vi "FGV_Dictionnaire.vi"(6 "FichierDictionnaire":path, 7 "Command":T3, 8 "error in (no error)":errorcluster, 9 "Dictionnaire In":T1, 10 "Chaîne":string, 11 "Clé":string) -> (0 "error out":errorcluster, 1 "Dictionnaire Out":T1, 3 "Traduction":string)   [LabVIEW 2011]
uses:
  EnumCommandDictionnaire.ctl
  Dictionnaire.ctl
  CleValeur.ctl
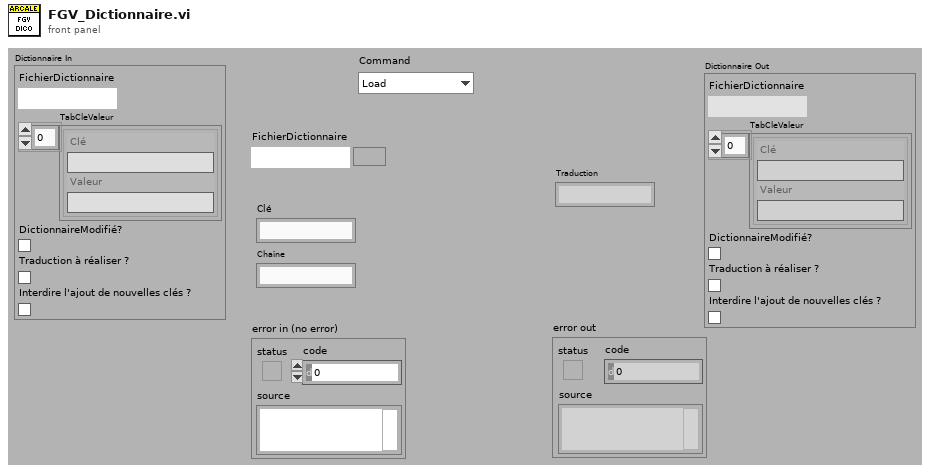
[diagram p1: front panel]
types:
  T1 = typedef "Dictionnaire.ctl" = cluster{"FichierDictionnaire":path, "TabCleValeur":T2[], "DictionnaireModifié?":bool, "Traduction à réaliser ?":bool, "Interdire l'ajout de nouvelles clés ?":bool}
  T2 = typedef "CleValeur.ctl" = cluster{"Clé":string, "Valeur":string}
  T3 = typedef "EnumCommandDictionnaire.ctl" = enum16{"Load", "Translate", "Save", "GetDico", "Set : A traduire = Vrai", "Set : A Traduire = Faux", "SetDico"}
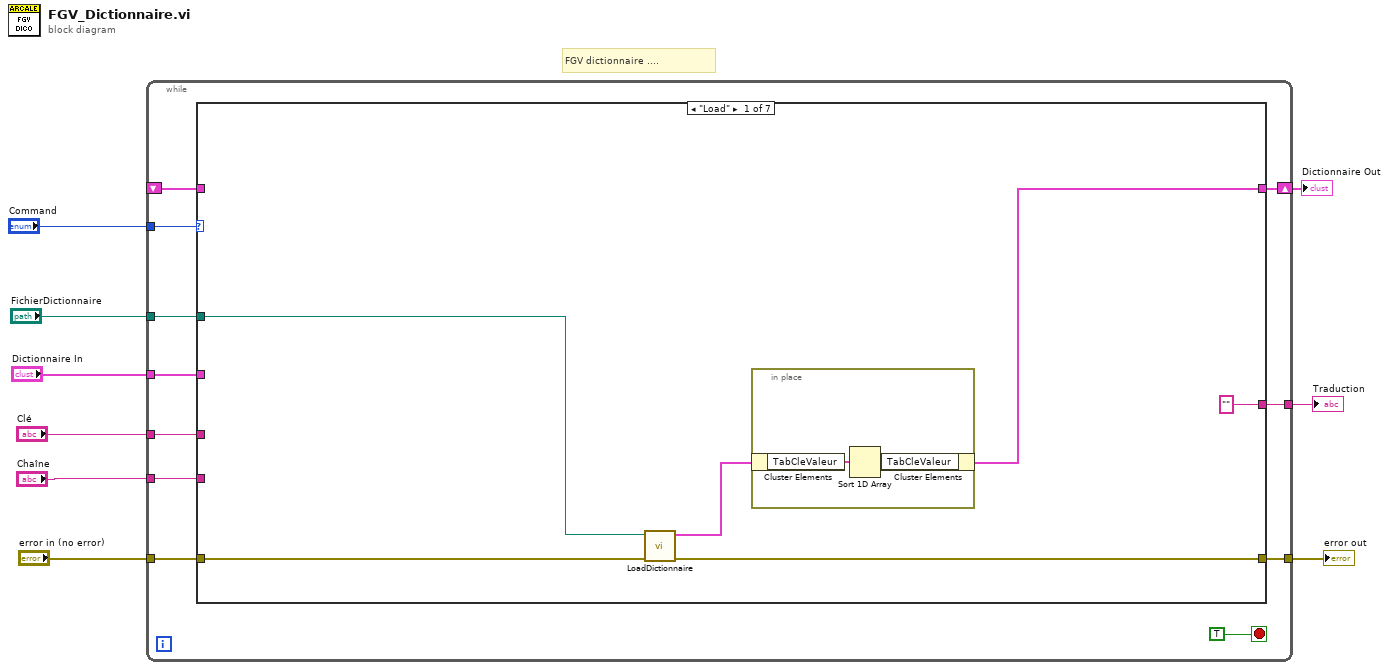
[diagram p0: block diagram]
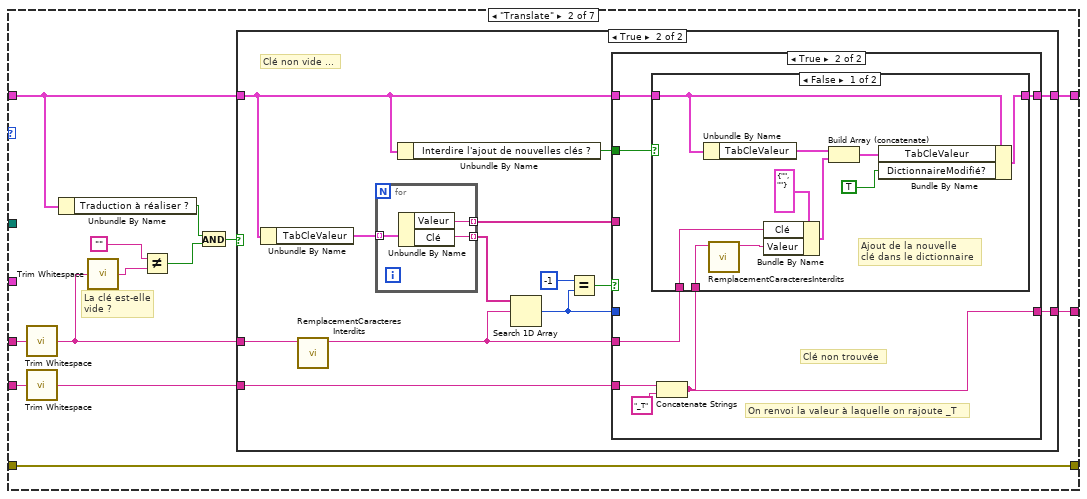
[diagram p2: hidden frame]
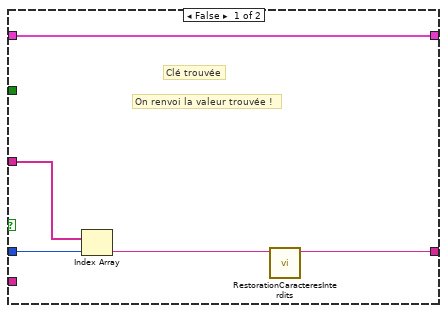
[diagram p4: hidden frame]
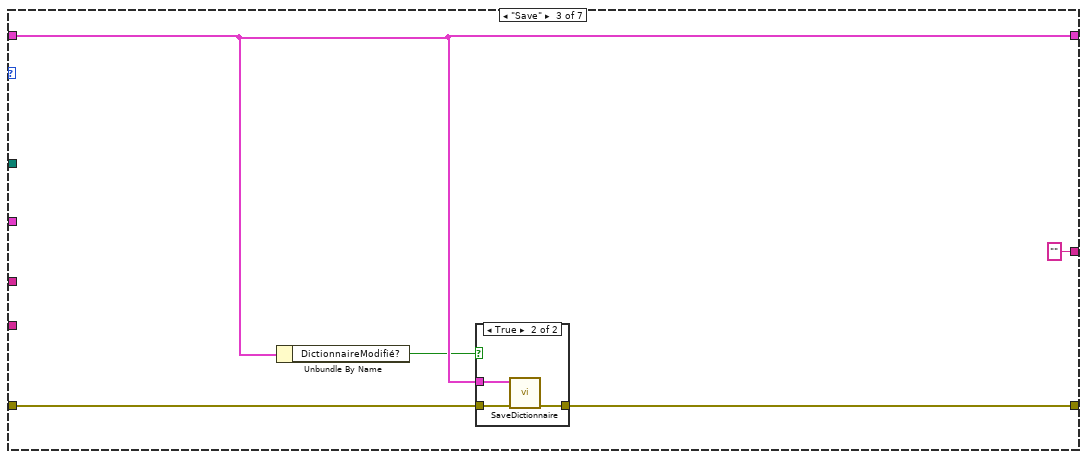
[diagram p6: hidden frame]
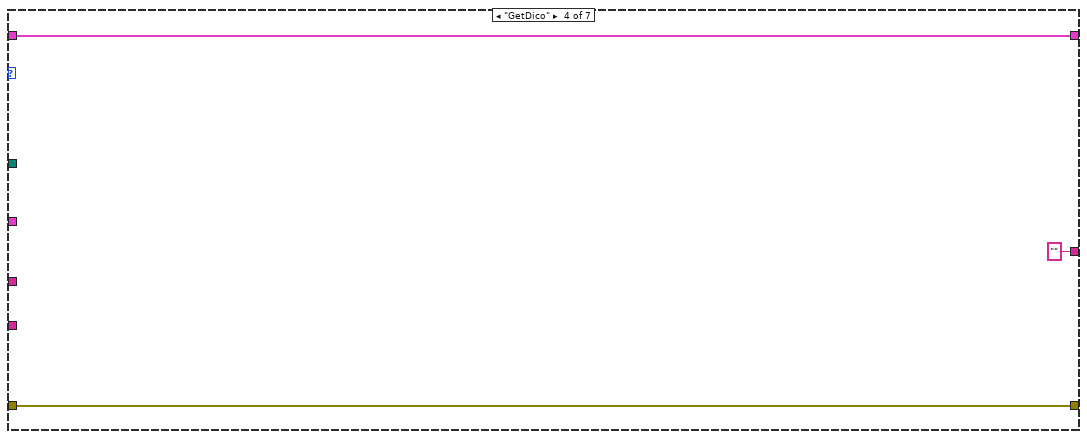
[diagram p8: hidden frame]
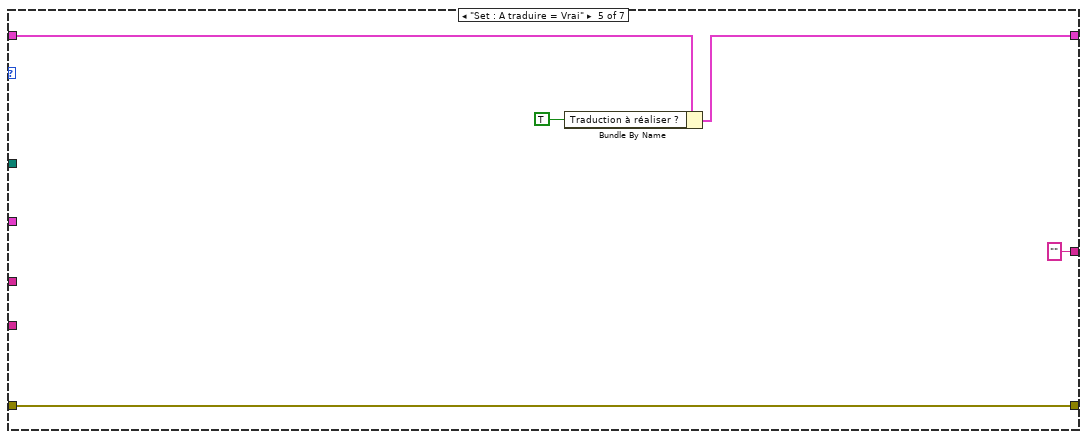
[diagram p9: hidden frame]
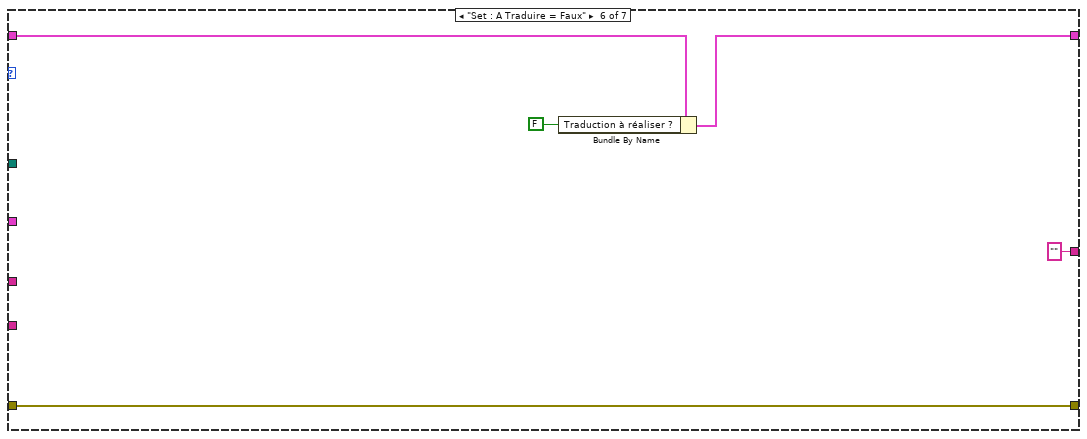
[diagram p10: hidden frame]
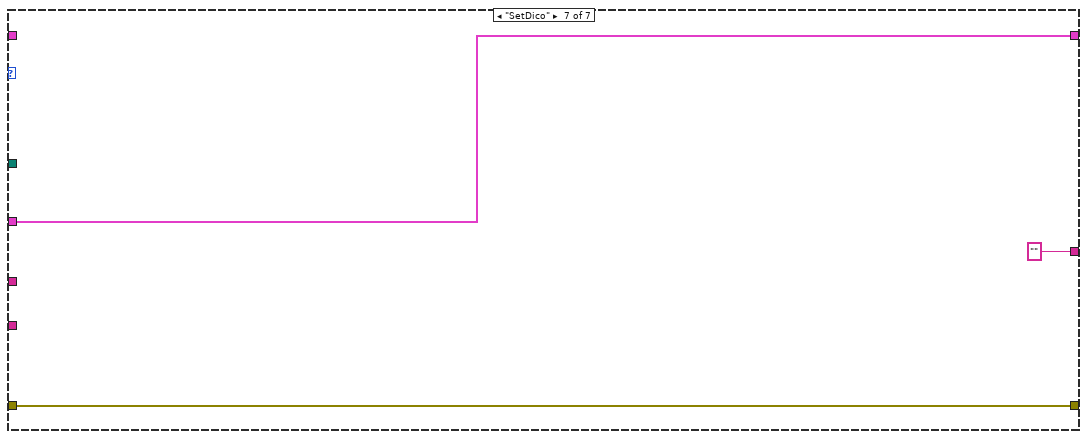
[diagram p11: hidden frame]
diagram:
  # "FGV dictionnaire ...."
  n1 = while {
    tunnel: "Command" -> [w19]
    shift-right: [w18] -> w2
    shift-left: _ -> [w17]
    tunnel: "error in (no error)" -> [w16]
    tunnel: [w15] -> w7
    tunnel: "Clé" -> [w14]
    tunnel: "Chaîne" -> [w13]
    tunnel: [w12] -> w4
    tunnel: "FichierDictionnaire" -> [w11]
    tunnel: "Dictionnaire In" -> [w10]
    stop <- TRUE stop-if-true
    n2 = case shown="\"Load\"" w19 {
      tunnel: [w21 w39 w84 w94 w97 w102 w107] -> w18
      tunnel: w17 -> [_ w36 w84 w94 w99 w103 _]
      tunnel: w16 -> [w25 w41 w86 w92 w96 w100 w106]
      tunnel: [w24 w41 w85 w92 w96 w100 w106] -> w15
      tunnel: w14 -> [_ w30 _ _ _ _ _]
      tunnel: w13 -> [_ w32 _ _ _ _ _]
      tunnel: ["" ("Valeur") w40 "" ("Valeur") "" ("Valeur") "" ("Valeur") "" ("Valeur") "" ("Valeur")] -> w12
      tunnel: w11 -> [w23 _ _ _ _ _ _]
      tunnel: w10 -> [_ _ _ _ _ _ w107]
      frame "Load" {
        n3 = call "LoadDictionnaire.vi"("error in (no error)"=w25, "FichierDictionnaire"=w23) -> ("error out"=w24:errorcluster, "Dictionnaire"=w22:T1)  [unwired: 8 in]
        n4 = in-place {
          n5 = in-place-cluster #1(w22) -> ("TabCleValeur"=w28:T2[])
          n6 = Sort 1D Array(array=w28) -> (sorted array=w27:T2[])
          n7 = in-place-cluster #1("TabCleValeur"=w27) -> (w21:T1)
        }
      }
      frame "Translate" {
        # "La clé est-elle\nvide ?"
        n8 = call <vilib>:"Trim Whitespace.vi"("string"=w30) -> ("trimmed string"=w29:string)  [unwired: 1 in]
        n9 = call <vilib>:"Trim Whitespace.vi"("string"=w32) -> ("trimmed string"=w31:string)  [unwired: 1 in]
        n10 = Unbundle By Name(w36) -> ("Traduction à réaliser ?"=w35:bool)
        n11 = call <vilib>:"Trim Whitespace.vi"("string"=w29) -> ("trimmed string"=w38:string)  [unwired: 1 in]
        n12 = Not Equal?(x="", y=w38) -> (x != y?=w34:bool)
        n13 = And(x=w35, y=w34) -> (x .and. y?=w33:bool)
        n14 = case shown="True" w33 {
          tunnel: w31 -> [w42 w46]
          tunnel: [w42 w50] -> w40
          tunnel: [w43 w49] -> w39
          tunnel: w36 -> [w43 w45]
          tunnel: w29 -> [_ w48]
          frame False {
            # "La traduction n'est pas à réaliser  ..."
          }
          frame True {
            # "Clé non vide ..."
            n15 = Unbundle By Name(w45) -> ("TabCleValeur"=w56:T2[])
            n16 = call "RemplacementCaracteresInterdits.vi"("String In"=w48) -> ("String Out"=w47:string)  [unwired: 9 in, 1 out]
            n17 = for {
              tunnel: w56 -> [w82] mode=indexing
              tunnel: [w81] -> w55 mode=indexing
              tunnel: [w80] -> w52 mode=indexing
              n18 = Unbundle By Name(w82) -> ("Valeur"=w80:string, "Clé"=w81:string)
            }
            n19 = Unbundle By Name(w45) -> ("Interdire l'ajout de nouvelles clés ?"=w44:bool)
            n20 = Search 1D Array(1D array=w55, element=w47) -> (index of element=w51:i32)  [unwired: 1 in]
            n21 = Equal?(x=-1, y=w51) -> (x = y?=w53:bool)
            n22 = case shown="True" w53 {
              tunnel: w46 -> [_ w64]
              tunnel: w52 -> [w61 _]
              tunnel: w51 -> [w60 _]
              tunnel: [w57 w63] -> w50
              tunnel: w45 -> [w59 w67]
              tunnel: w47 -> [_ w68]
              tunnel: [w59 w66] -> w49
              tunnel: w44 -> [_ w62]
              frame False {
                # "On renvoi la valeur trouvée !"
                # "Clé trouvée"
                n23 = Index Array(array=w61, index=w60) -> (element=w58:string)
                n24 = call "RestorationCaracteresInterdits.vi"("String In"=w58) -> ("String Out"=w57:string)  [unwired: 9 in, 1 out]
              }
              frame True {
                # "On renvoi la valeur à laquelle on rajoute _T"
                # "Clé non trouvée"
                n25 = Concatenate Strings(w64, "_T" ("string")) -> (w63:string)
                n26 = case shown="False" w62 {
                  tunnel: w68 -> [w75 _]
                  tunnel: w67 -> [w73 w79]
                  tunnel: [w72 w79] -> w66
                  tunnel: w63 -> [w70 _]
                  frame False {
                    # "Ajout de la nouvelle\nclé dans le dictionnaire"
                    n27 = Unbundle By Name(w73) -> ("TabCleValeur"=w78:T2[])
                    n28 = call "RemplacementCaracteresInterdits.vi"("String In"=w70) -> ("String Out"=w69:string)  [unwired: 9 in, 1 out]
                    n29 = Bundle By Name(cluster=T2 {"Clé"="", "Valeur"=""} ("CléValeur"), "Clé"=w75, "Valeur"=w69) -> (w76:T2)
                    n30 = Build Array (concatenate)(w78, w76) -> (w74:T2[])
                    n31 = Bundle By Name(cluster=w73, "TabCleValeur"=w74, "DictionnaireModifié?"=TRUE) -> (w72:T1)
                  }
                  frame True {
                    # "Interdiction d'ajouter de nouvelles clés au\ndictionnaire ..."
                  }
                }
              }
            }
          }
        }
      }
      frame "Save" {
        n32 = Unbundle By Name(w84) -> ("DictionnaireModifié?"=w83:bool)
        n33 = case shown="True" w83 {
          tunnel: w86 -> [w88 w91]
          tunnel: [w88 w90] -> w85
          tunnel: w84 -> [_ w89]
          frame False {
          }
          frame True {
            n34 = call "SaveDictionnaire.vi"("error in (no error)"=w91, "Dictionnaire"=w89) -> ("error out"=w90:errorcluster)  [unwired: 9 in]
          }
        }
      }
      frame "GetDico" {
      }
      frame "Set : A traduire = Vrai" {
        n35 = Bundle By Name(cluster=w99, "Traduction à réaliser ?"=TRUE) -> (w97:T1)
      }
      frame "Set : A Traduire = Faux" {
        n36 = Bundle By Name(cluster=w103, "Traduction à réaliser ?"=FALSE) -> (w102:T1)
      }
      frame "SetDico" {
      }
    }
  }
  "error out" <- w7
  "Traduction" <- w4
  "Dictionnaire Out" <- w2
